vi "Master Setup Import.vi"(6 "Sorted Titles Indices":i32[](array[numeric]), 9 "Sorted Titles":string[](array[string]), 10 "Master Setup Path In":path, 11 "Master Setup In":path[](array[path])) -> (1 "Cancelled":bool, 2 "Master Setup Path Out":path, 3 "Master Setup Out":path[](array[path]))   [LabVIEW 2017]
uses:
  <vilib>/zip/NI_Unzip.lvlib
panel:
  out "Master Setup Assorted 2":path[](array[path])
  out "Tab Control":enum32{"Select Files", "Confirm Import"}(tab)
  in  "Files Available":i32[](listbox)
  in  "Files to Import":i32(listbox)
  in  "Remove":bool
  in  "Add":bool
  in  "Import":bool
  in  "Cancel":bool
  in  "Select File to Import From":path
  in  "Ok":bool
  in  "Cancel2":bool
  in  "Import All":bool
  in  "Auto Correct":bool
  out "Status":u16[](array[ring])
  out "Setup Files":string[](array[string])
  out "Target File Paths":path[](array[path])
  in  "Browse":bool[](array[boolean])
  # "REPS Import Setup Utility"
  # "File already Exists in the target path"
  # "File Path Ok"
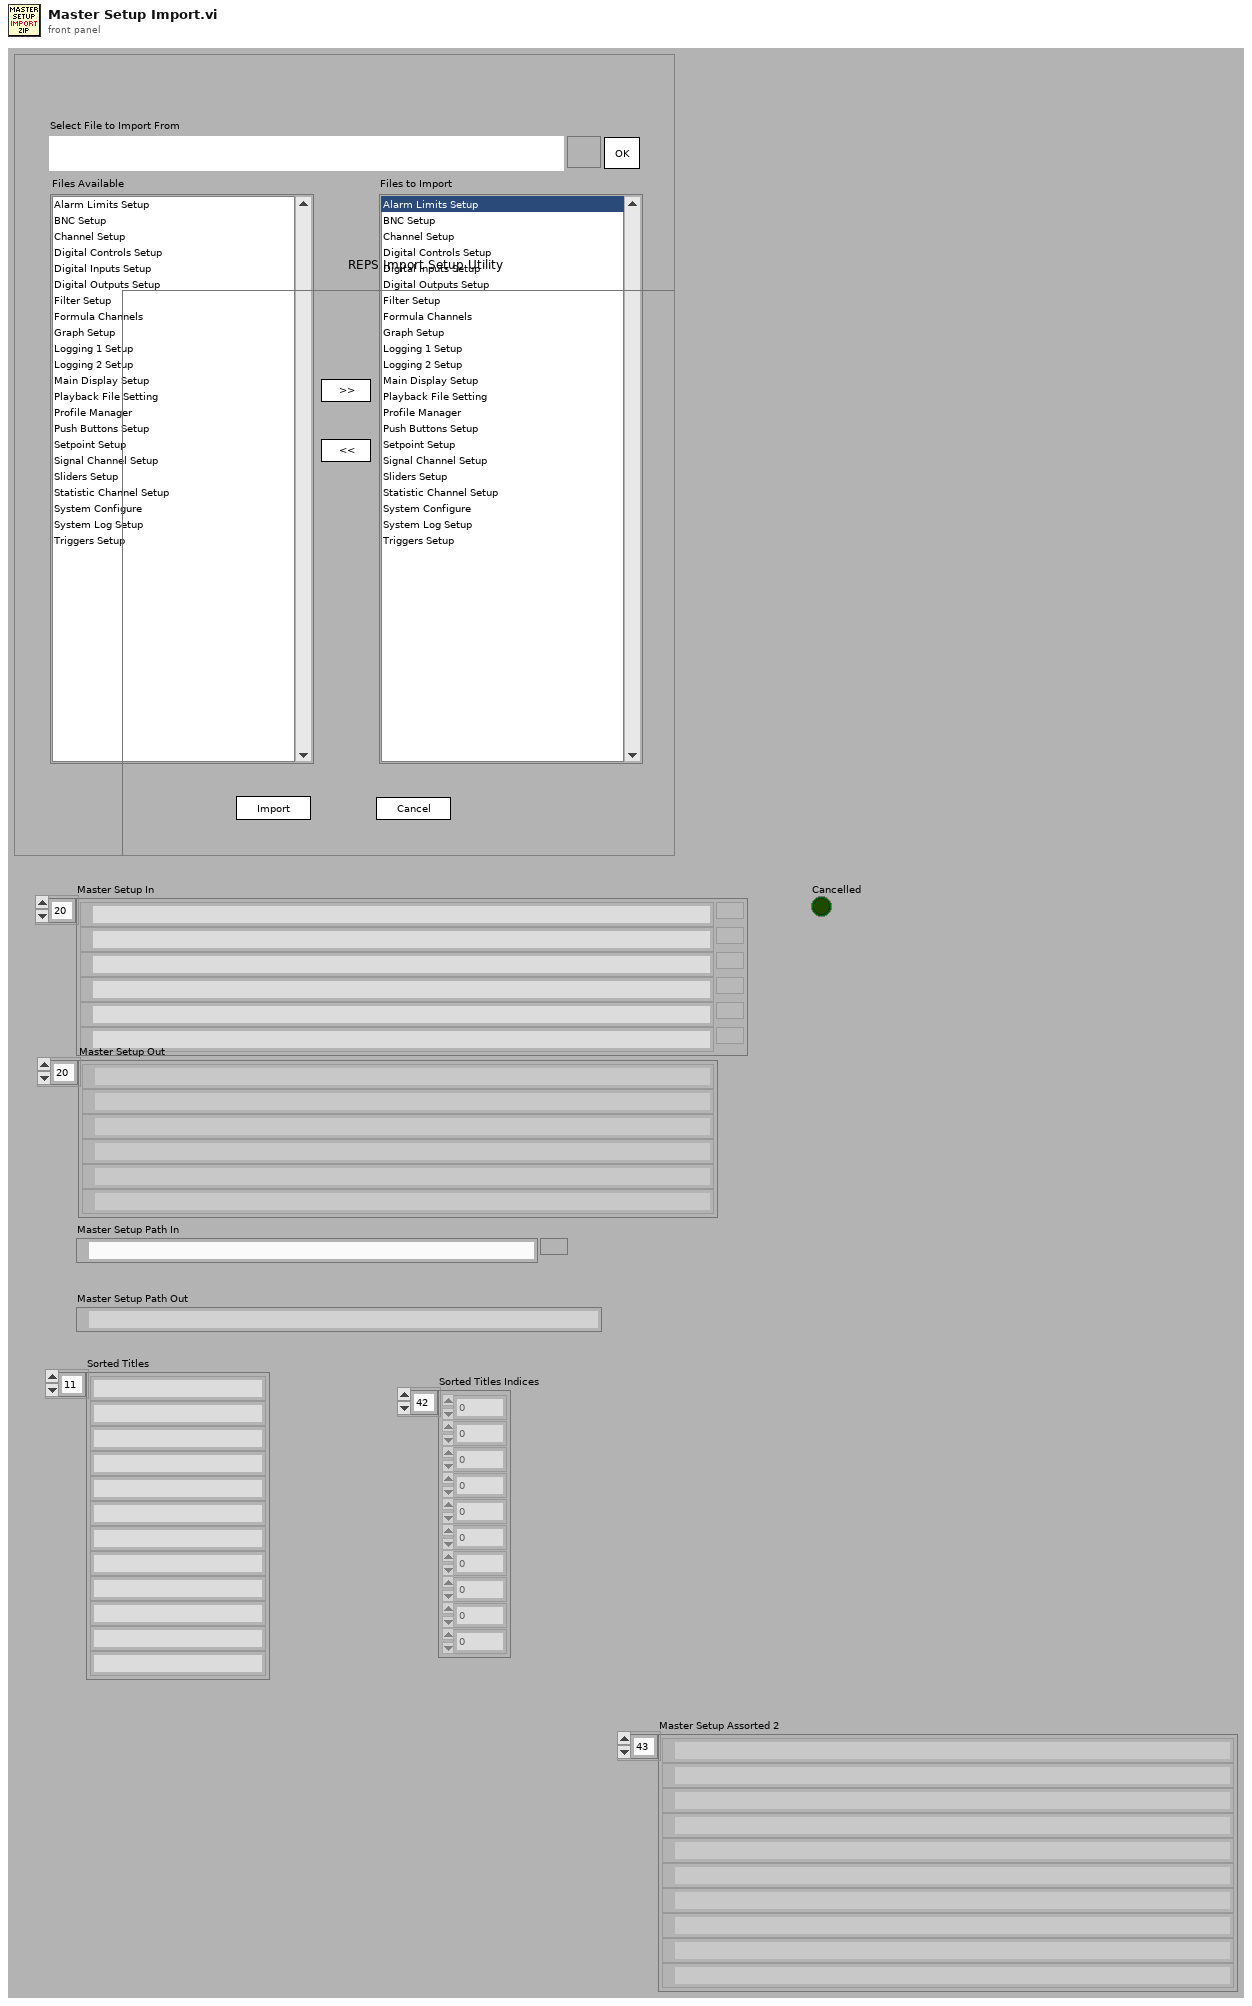
[diagram p1: front panel]
types:
  T1 = enum16{"<Init>", "<Poll>", "<Preview>", "<CheckFiles>", "<PopulateListBox>", "<ImportAddFile>", "<ImportRemoveFile>", "<Import>", "<CheckIfFileExists>", "<CopyFiles>", "<ConfirmOverwrite>", "<BrowseNewFile>", "<AutoCorrect>", "<Exit>"}
  T2 = enum32{"invalid app kind", "Development System", "Run Time System", "Student Edition", "Embedded LabVIEW", "Evaluation", "Custom"}
  T3 = enum8{"Enabled", "Disabled", "Disabled and Grayed Out"}
  T4 = cluster{"Preview files":path[], "Preview Folder":path, "File Types":string[], "Import files":path[], "Import File Types":string[], "Target files":path[], "Actual File Paths":path[], "vi reference":refnum<vi>, path[], "Sorted Titles":string[], i32[]}
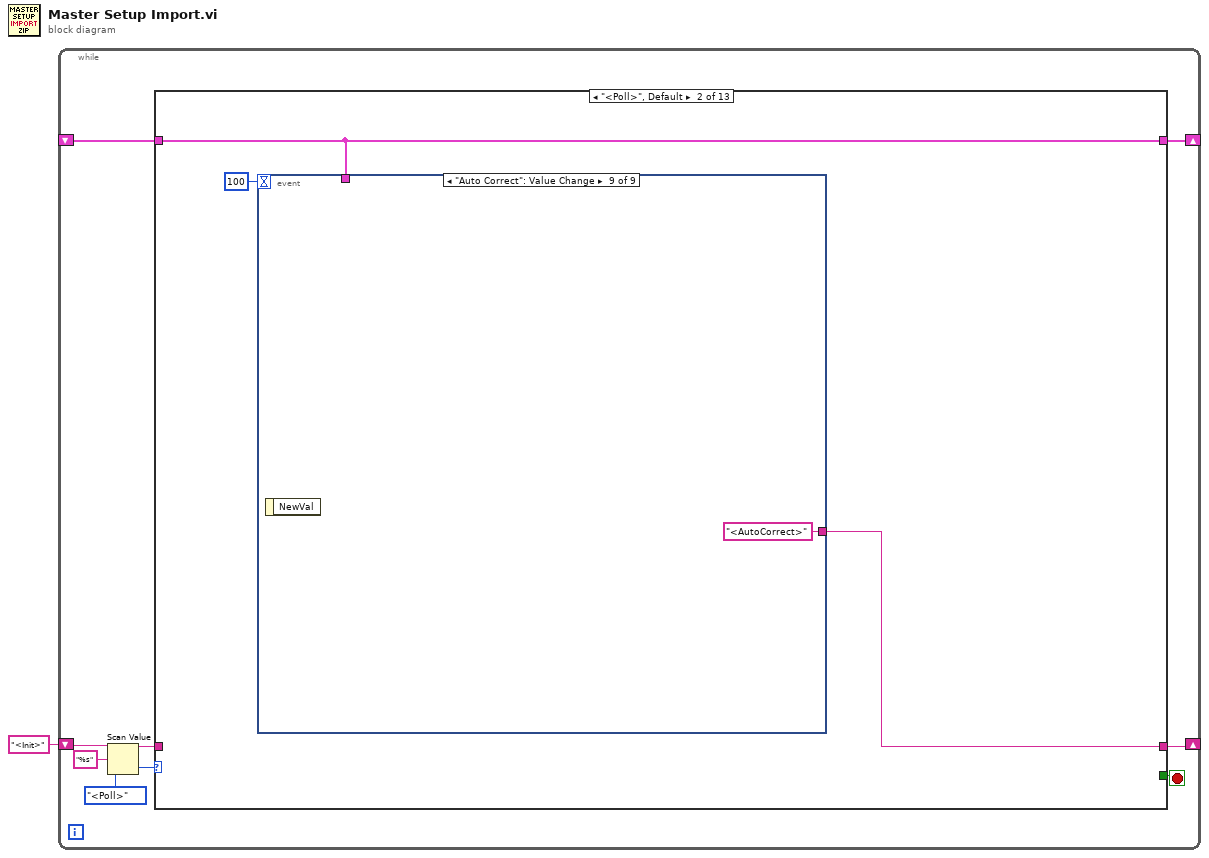
[diagram p0: block diagram]
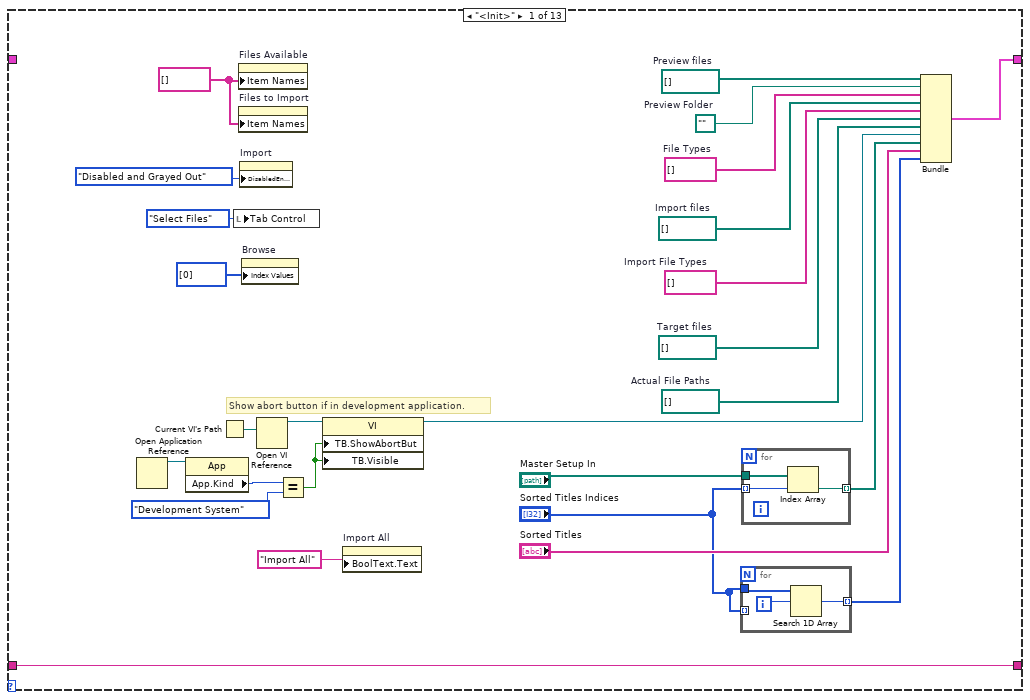
[diagram p2: hidden frame]
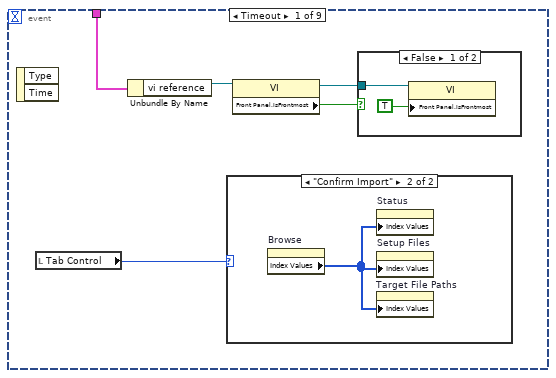
[diagram p3: hidden frame]
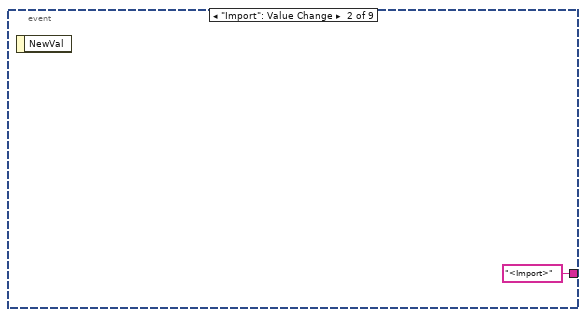
[diagram p6: hidden frame]
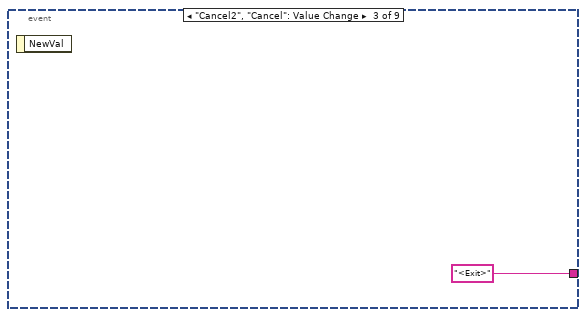
[diagram p7: hidden frame]
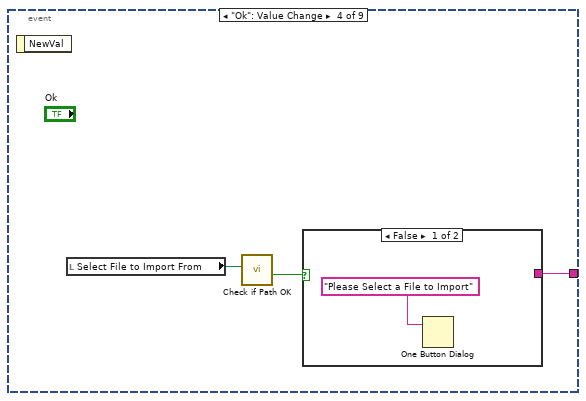
[diagram p8: hidden frame]
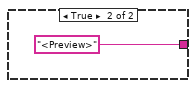
[diagram p9: hidden frame]
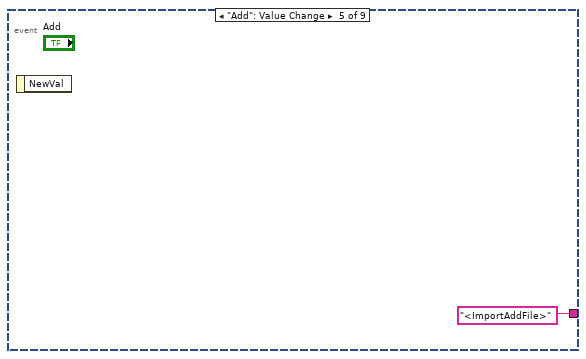
[diagram p10: hidden frame]
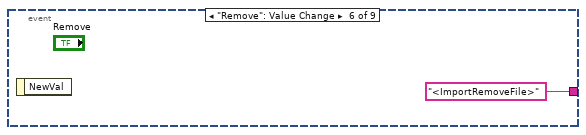
[diagram p11: hidden frame]
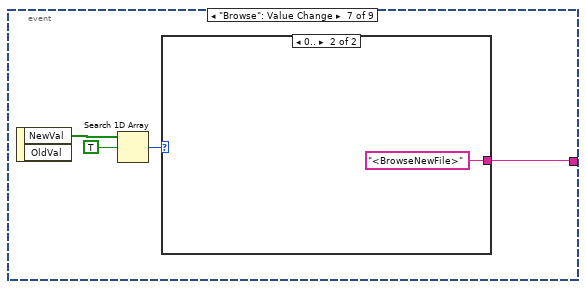
[diagram p12: hidden frame]
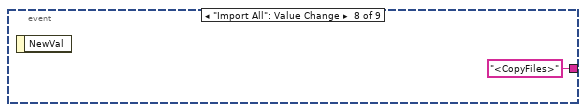
[diagram p14: hidden frame]
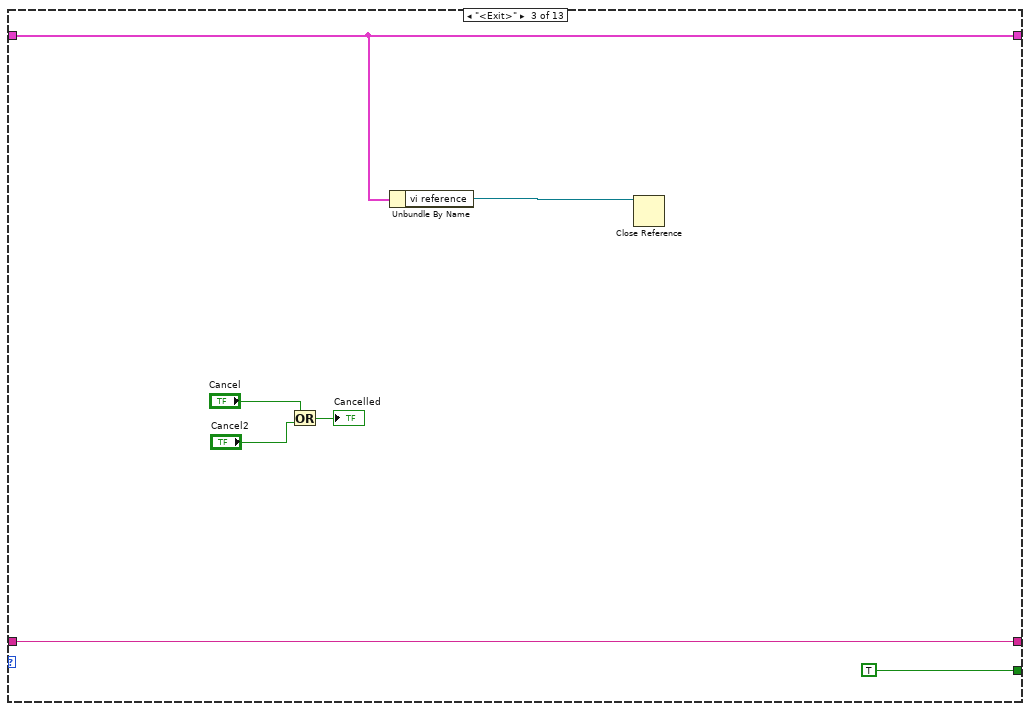
[diagram p15: hidden frame]
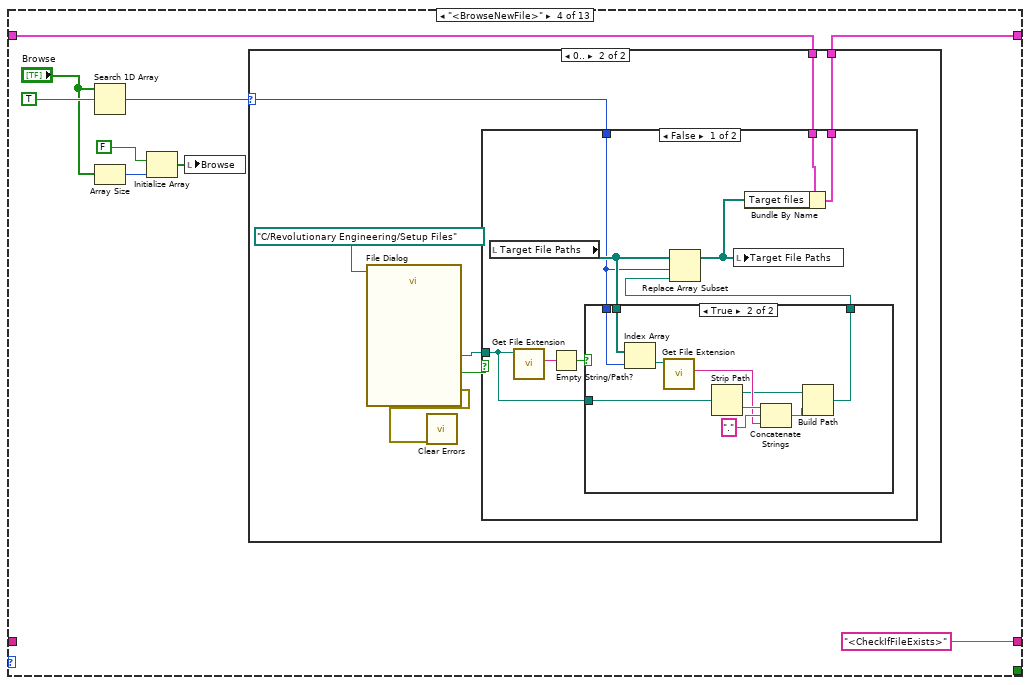
[diagram p16: hidden frame]
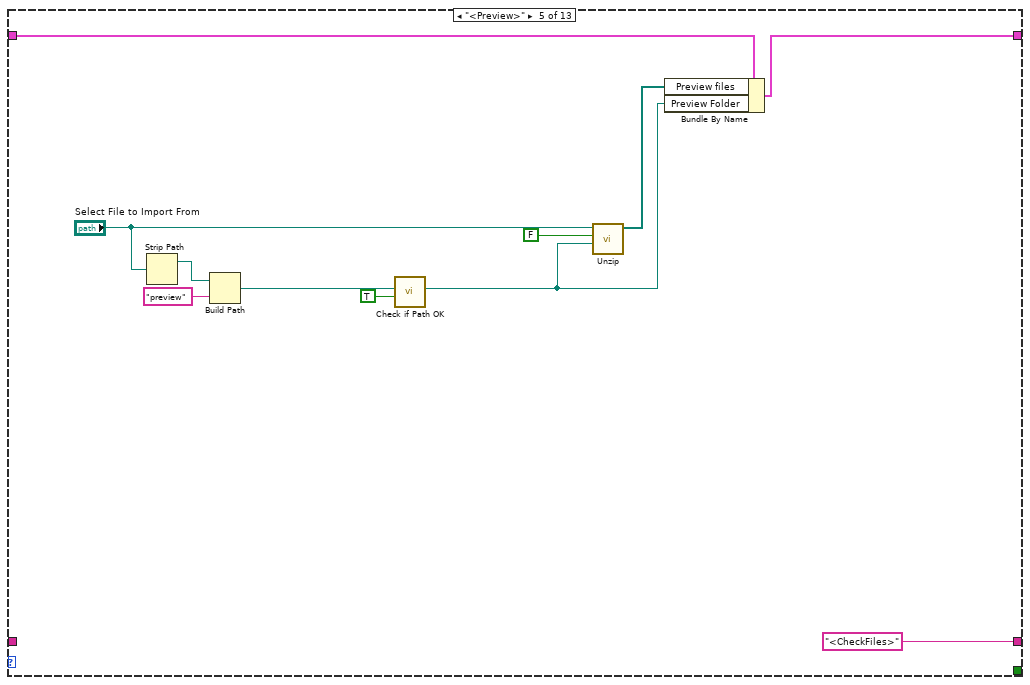
[diagram p20: hidden frame]
diagram:
  n1 = while {
    shift-right: [w8] -> _
    shift-left: "<Init>" -> [w10]
    shift-right: [w4] -> _
    shift-left: _ -> [w3]
    stop <- w5 stop-if-true
    n2 = Scan Value(string=w10, format string="%s", default (0 dbl)=T1."<Poll>") -> (output string=w9:string, value=w6:T1)
    n3 = case shown="\"<Poll>\", Default" w6 {
      tunnel: w9 -> [w34 _ w76 _ _ _ w157 w160 w180 _ _ _ _]
      tunnel: [w34 w44 w76 "<CheckIfFileExists>" "<CheckFiles>" w126 w157 w160 w180 "<CheckIfFileExists>" w220 "<Exit>" "<CheckIfFileExists>"] -> w8
      tunnel: [_ _ TRUE _ _ _ FALSE _ _ _ _ _ _] -> w5
      tunnel: [w33 w43 w74 w82 w122 w131 w147 w159 w181 w184 w224 w242 w278] -> w4
      tunnel: w3 -> [_ w43 w74 w83 w124 w131 w148 w159 w181 w185 w224 w242 w279]
      frame "<Init>" {
        w25 = path[] []  # Actual File Paths
        w26 = path[] []  # Target files
        w28 = string[] []  # Import File Types
        w29 = path[] []  # Import files
        w30 = string[] []  # File Types
        w31 = path ""  # Preview Folder
        w32 = path[] []  # Preview files
        w36 = string[] [] ("Item Names")
        # "Show abort button if in development application."
        n4 = Open Application Reference() -> (3:w24:refnum<vi>)  [unwired: 4 in, 1 out]
        n5 = property class="App"(reference=w24) -> ("App.Kind"=w23:T2)  [unwired: 1 in, 2 out]
        n6 = Current VI's Path() -> (path=w22:path)
        n7 = local write "Tab Control"(enum32{"Select Files", "Confirm Import"}."Select Files" ("Tab Control")) -> ()
        n8 = property on="Files Available" class="LstBox (strict)"("Item Names"=w36) -> ()  [unwired: 2 in, 2 out]
        n9 = property on="Files to Import" class="LstBox (strict)"("Item Names"=w36) -> ()  [unwired: 2 in, 2 out]
        n10 = property on="Import" class="Bool"("DisabledEnum"=T3."Disabled and Grayed Out" ("Disabled")) -> ()  [unwired: 2 in, 2 out]
        n11 = property on="Browse" class="Arr"("Index Values"=u32[] [0]) -> ()  [unwired: 2 in, 2 out]
        n12 = Open VI Reference(vi path=w22) -> (vi reference=w21:refnum<vi>)  [unwired: 5 in, 1 out]
        n13 = Equal?(x=w23, y=T2."Development System" ("Application:Kind")) -> (x = y?=w20:bool)
        n14 = property class="VI"(reference=w21, "TB.ShowAbortBut"=w20, "TB.Visible"=w20) -> (reference out=w18:refnum<vi>)  [unwired: 1 in, 1 out]
        n15 = property on="Import All" class="Bool"("BoolText.Text"="Import All" ("Label.Text")) -> ()  [unwired: 2 in, 2 out]
        n16 = for {
          tunnel: "Sorted Titles Indices" -> [w39]
          tunnel: "Sorted Titles Indices" -> [_] mode=indexing
          tunnel: [w37] -> w14 mode=indexing
          i -> [w38]
          n17 = Search 1D Array(1D array=w39, element=w38) -> (index of element=w37:i32)  [unwired: 1 in]
        }
        n18 = for {
          tunnel: "Master Setup In" -> [w42]
          tunnel: "Sorted Titles Indices" -> [w40] mode=indexing
          tunnel: [w41] -> w17 mode=indexing
          n19 = Index Array(array=w42, index=w40) -> (element=w41:path)
        }
        n20 = Bundle("Preview files"=w32, "Preview Folder"=w31, "File Types"=w30, "Import files"=w29, "Import File Types"=w28, "Target files"=w26, "Actual File Paths"=w25, "vi reference"=w18, w17, "Sorted Titles"="Sorted Titles", w14) -> (w33:T4)  [unwired: 1 in]
      }
      frame "<Poll>", Default {
        n21 = event shown="[8] \"Auto Correct\": Value Change" {
          selector: _ -> [_ _ _ _ _ _ _ _ _]
          dyn-events: _ -> [_ _ _ _ _ _ _ _ _]
          timeout: 100 -> [_ _ _ _ _ _ _ _ _]
          tunnel: [_ "<Import>" "<Exit>" w58 "<ImportAddFile>" "<ImportRemoveFile>" w63 "<CopyFiles>" "<AutoCorrect>"] -> w44
          tunnel: w43 -> [w49 _ _ _ _ _ _ _ _]
          event Timeout {
            n22 = event-data() -> ()  [unwired: 1 in, 2 out]
            n23 = local read "Tab Control"() -> (w50:enum32{"Select Files", "Confirm Import"})
            n24 = Unbundle By Name(w49) -> ("vi reference"=w48:refnum<vi>)
            n25 = case shown="\"Confirm Import\"" w50 {
              frame "Select Files", Default {
              }
              frame "Confirm Import" {
                n26 = property on="Browse" class="Arr"() -> ("Index Values"=w53:u32[])  [unwired: 2 in, 2 out]
                n27 = property on="Status" class="Arr (strict)"("Index Values"=w53) -> ()  [unwired: 2 in, 2 out]
                n28 = property on="Setup Files" class="Arr (strict)"("Index Values"=w53) -> ()  [unwired: 2 in, 2 out]
                n29 = property on="Target File Paths" class="Arr (strict)"("Index Values"=w53) -> ()  [unwired: 2 in, 2 out]
              }
            }
            n30 = property class="VI"(reference=w48) -> (reference out=w46:refnum<vi>, "Front Panel.IsFrontmost"=w47:bool)  [unwired: 1 in, 1 out]
            n31 = case shown="False" w47 {
              tunnel: w46 -> [w52 _]
              frame False {
                n32 = property class="VI"(reference=w52, "Front Panel.IsFrontmost"=TRUE ("Front Panel Window:Is Frontmost")) -> ()  [unwired: 1 in, 2 out]
              }
              frame True {
              }
            }
          }
          event "Import": Value Change {
            n33 = event-data() -> ()  [unwired: 1 in, 1 out]
          }
          event "Cancel2", "Cancel": Value Change {
            n34 = event-data() -> ()  [unwired: 1 in, 1 out]
          }
          event "Ok": Value Change {
            n35 = event-data() -> ()  [unwired: 1 in, 1 out]
            n36 = local read "Select File to Import From"() -> (w57:path)
            n37 = call "Check if Path OK.vi"("Path"=w57) -> ("Path OK"=w56:bool)  [unwired: 8 in, 2 out]
            n38 = case shown="False" w56 {
              tunnel: [_ "<Preview>"] -> w58
              frame False {
                n39 = One Button Dialog(message="Please Select a File to Import") -> ()  [unwired: 1 in, 1 out]
              }
              frame True {
              }
            }
          }
          event "Add": Value Change {
            n40 = event-data() -> ()  [unwired: 1 in, 1 out]
          }
          event "Remove": Value Change {
            n41 = event-data() -> ()  [unwired: 1 in, 1 out]
          }
          event "Browse": Value Change {
            n42 = event-data() -> ("NewVal"=w66:bool[])  [unwired: 1 in, 1 out]
            n43 = Search 1D Array(1D array=w66, element=TRUE) -> (index of element=w64:i32)  [unwired: 1 in]
            n44 = case shown="0.." w64 {
              tunnel: [_ "<BrowseNewFile>"] -> w63
              frame ..-1 {
              }
              frame 0.. {
              }
            }
          }
          event "Import All": Value Change {
            n45 = event-data() -> ()  [unwired: 1 in, 1 out]
          }
          event "Auto Correct": Value Change {
            n46 = event-data() -> ()  [unwired: 1 in, 1 out]
          }
        }
      }
      frame "<Exit>" {
        n47 = Or(x="Cancel", y="Cancel2") -> (x .or. y?=→"Cancelled":bool)
        n48 = Unbundle By Name(w74) -> ("vi reference"=w73:refnum<vi>)
        n49 = Close Reference(reference=w73) -> ()  [unwired: 1 in, 1 out]
      }
      frame "<BrowseNewFile>" {
        n50 = Search 1D Array(1D array="Browse", element=TRUE) -> (index of element=w84:i32)  [unwired: 1 in]
        n51 = Array Size(array="Browse") -> (size(s)=w80:i32)
        n52 = Initialize Array(FALSE ("element"), w80) -> (w78:bool[])
        n53 = local write "Browse"(w78) -> ()
        n54 = case shown="0.." w84 {
          selector: w84 -> [_ w90]
          tunnel: w83 -> [w86 w89]
          tunnel: [w86 w88] -> w82
          frame Default {
          }
          frame 0.. {
            n55 = call "File Dialog"("start path"=path "C:/Revolutionary Engineering/Setup Files") -> ("selected path"=w91:path, "cancelled"=w92:bool, "error out"=w87:errorcluster)  [unwired: 11 in, 1 out]
            n56 = call <vilib>:"Clear Errors.vi"("error in (no error)"=w87) -> ()  [unwired: 5 in, 2 out]
            n57 = case shown="False" w92 {
              tunnel: w91 -> [w95 _]
              tunnel: w90 -> [w96 _]
              tunnel: w89 -> [w102 w114]
              tunnel: [w101 w114] -> w88
              frame False {
                n58 = local read "Target File Paths"() -> (w97:path[])
                n59 = call <vilib>:"Get File Extension.vi"("file"=w95) -> ("lowercase file extension"=w99:string)  [unwired: 6 in, 4 out]
                n60 = Empty String/Path?(string/path=w99) -> (empty?=w98:bool)
                n61 = case shown="True" w98 {
                  tunnel: w97 -> [_ w113]
                  tunnel: w96 -> [_ w112]
                  tunnel: w95 -> [w103 w110]
                  tunnel: [w103 w104] -> w94
                  frame False {
                  }
                  frame True {
                    n62 = Index Array(array=w113, index=w112) -> (element=w111:path)
                    n63 = call <vilib>:"Get File Extension.vi"("file"=w111) -> ("lowercase file extension"=w107:string)  [unwired: 6 in, 4 out]
                    n64 = Strip Path(path=w110) -> (stripped path=w106:path, name=w109:string)
                    n65 = Concatenate Strings(w109, ".", w107) -> (w105:string)
                    n66 = Build Path(base path=w106, name or relative path=w105) -> (appended path=w104:path)
                  }
                }
                n67 = Replace Array Subset(array=w97, new element=w94, index=w96) -> (w100:path[])
                n68 = local write "Target File Paths"(w100) -> ()
                n69 = Bundle By Name(cluster=w102, "Target files"=w100) -> (w101:T4)
              }
              frame True {
              }
            }
          }
        }
      }
      frame "<Preview>" {
        n70 = Strip Path(path="Select File to Import From") -> (stripped path=w125:path)  [unwired: 1 out]
        n71 = Build Path(base path=w125, name or relative path="preview") -> (appended path=w116:path)
        n72 = call "Check if Path OK.vi"("Create if not found? (F)"=TRUE, "Path"=w116) -> ("Path"=w115:path)  [unwired: 7 in, 2 out]
        n73 = call <vilib>:"Unzip.vi"("Target directory (same as Zip file if empty)"=w115, "Preview only?"=FALSE, "Zip file"="Select File to Import From") -> ("Unzipped files"=w123:path[])  [unwired: 6 in, 2 out]
        n74 = Bundle By Name(cluster=w124, "Preview files"=w123, "Preview Folder"=w115) -> (w122:T4)
      }
      frame "<CheckFiles>" {
        n75 = Unbundle By Name(w131) -> ("Preview Folder"=w130:path)
        n76 = List Folder(path=w130) -> (filenames=w129:string[])  [unwired: 3 in, 3 out]
        n77 = Search 1D Array(1D array=w129, element="repsexport.txt") -> (index of element=w127:i32)  [unwired: 1 in]
        n78 = case shown="..-1" w127 {
          tunnel: ["<PopulateListBox>" "<Poll>"] -> w126
          frame 0.. {
            # "Valid REPS Export File"
            n79 = property on="Import" class="Bool"("DisabledEnum"=T3."Enabled" ("Disabled")) -> ()  [unwired: 2 in, 2 out]
          }
          frame ..-1 {
            # "Invalid REPS Export File"
            n80 = One Button Dialog(message="Invalid REPS Import File") -> ()  [unwired: 1 in, 1 out]
          }
        }
      }
      frame "<PopulateListBox>" {
        w140 = string[] []
        w138 = "," ("delimiter (Tab)")
        w139 = "%s" ("format string")
        n81 = Unbundle By Name(w148) -> ("Preview Folder"=w151:path)
        n82 = Build Path(base path=w151, name or relative path="repsexport.txt" ("element")) -> (appended path=w150:path)
        n83 = Open/Create/Replace File(file path (use dialog)=w150) -> (refnum out=w154:refnum<file>, error out=w155:errorcluster)  [unwired: 5 in, 1 out]
        n84 = Read from Text File(file (use dialog)=w154, error in=w155) -> (refnum out=w152:refnum<file>, text=w146:string, error out=w153:errorcluster)  [unwired: 2 in, 1 out]
        n85 = Close File(refnum=w152, error in=w153) -> ()  [unwired: 2 out]
        n86 = Match Pattern(string=w146, regular expression="REPS_File_Paths" ("string")) -> (before substring=w144:string, after substring=w143:string)  [unwired: 1 in, 2 out]
        n87 = Spreadsheet String To Array(delimiter (Tab)=w138, format string=w139, spreadsheet string=w144, array type (2D Dbl)=w140) -> (array=w137:string[])
        n88 = Spreadsheet String To Array(delimiter (Tab)=w138, format string=w139, spreadsheet string=w143, array type (2D Dbl)=w140) -> (array=w142:string[])
        n89 = for {
          tunnel: w137 -> [_] mode=indexing
          tunnel: [w158] -> w136 mode=indexing
          i -> [w158]
        }
        n90 = String To Path(string=w142) -> (path=w141:path[])
        n91 = property on="Files Available" class="LstBox (strict)"("Item Names"=w137, "Value"=w136) -> ()  [unwired: 2 in, 2 out]
        n92 = Bundle By Name(cluster=w148, "File Types"=w137, "Actual File Paths"=w141) -> (w147:T4)
      }
      frame "<ImportAddFile>" {
        n93 = property on="Files Available" class="LstBox (strict)"() -> ("Item Names"=w164:string[])  [unwired: 2 in, 2 out]
        n94 = property on="Files to Import" class="LstBox (strict)"() -> ("Item Names"=w162:string[])  [unwired: 2 in, 2 out]
        n95 = for {
          tunnel: "Files Available" -> [w169] mode=indexing
          tunnel: w164 -> [w170]
          shift-right: [w165] -> w161
          shift-left: w162 -> [w167]
          n96 = Index Array(array=w170, index=w169) -> (element=w166:string)
          n97 = Search 1D Array(1D array=w167, element=w166) -> (index of element=w168:i32)  [unwired: 1 in]
          n98 = case shown="..-1" w168 {
            tunnel: w167 -> [w171 w174]
            tunnel: w166 -> [_ w173]
            tunnel: [w171 w172] -> w165
            frame 0.. {
            }
            frame ..-1 {
              n99 = Build Array (concatenate)(w174, w173) -> (w172:string[])
            }
          }
        }
        n100 = property on="Files to Import" class="LstBox (strict)"("Item Names"=w161) -> ()  [unwired: 2 in, 2 out]
      }
      frame "<ImportRemoveFile>" {
        n101 = property on="Files to Import" class="LstBox (strict)"() -> ("Item Names"=w178:string[])  [unwired: 2 in, 2 out]
        n102 = Decrement(x="Files to Import") -> (x-1=w175:i32)
        n103 = Delete From Array(array=w178, length=1, index="Files to Import") -> (array with subset deleted=w177:string[])  [unwired: 1 out]
        n104 = local write "Files to Import"(w175) -> ()
        n105 = property on="Files to Import" class="LstBox (strict)"("Item Names"=w177) -> ()  [unwired: 2 in, 2 out]
      }
      frame "<Import>" {
        n106 = property on="Files to Import" class="LstBox (strict)"() -> ("Item Names"=w183:string[])  [unwired: 2 in, 2 out]
        n107 = Empty Array?(array=w183) -> (empty?=w182:bool)
        n108 = case shown="False" w182 {
          tunnel: w183 -> [w193 _]
          tunnel: w185 -> [w192 w205]
          tunnel: [w191 w205] -> w184
          frame False {
            n109 = Unbundle By Name(w192) -> ("Actual File Paths"=w189:path[], "Preview files"=w194:path[], "File Types"=w195:string[])
            n110 = for {
              tunnel: w193 -> [w203] mode=indexing
              tunnel: w195 -> [w200]
              tunnel: w194 -> [w202]
              tunnel: [w201] -> w190 mode=indexing
              tunnel: [w199] -> w187 mode=indexing
              tunnel: w189 -> [w198]
              tunnel: [w196] -> w188 mode=indexing
              n111 = Search 1D Array(1D array=w200, element=w203) -> (index of element=w197:i32)  [unwired: 1 in]
              n112 = Index Array(array=w198, index=w197) -> (element=w196:path)
              n113 = Index Array(array=w202, index=w197) -> (element=w201:path)
              n114 = Index Array(array=w200, index=w197) -> (element=w199:string)
            }
            n115 = Bundle By Name(cluster=w192, "Target files"=w188, "Import files"=w190, "Import File Types"=w187) -> (w191:T4)
          }
          frame True {
            n116 = One Button Dialog(message="No Files Selected for Import") -> ()  [unwired: 1 in, 1 out]
          }
        }
      }
      frame "<CheckIfFileExists>" {
        n117 = Unbundle By Name(w224) -> ("Target files"=w219:path[], "Import File Types"=w217:string[])
        "Target File Paths" <- w219
        "Setup Files" <- w217
        n118 = for {
          workers-P: _ -> [_]
          tunnel: w219 -> [w230] mode=indexing
          tunnel: [w228] -> w223 mode=indexing
          tunnel: [w225] -> w218 mode=indexing
          n119 = call "Check if Path OK.vi"("Create if not found? (F)"=FALSE, "Path"=w230) -> ("Path OK"=w228:bool)  [unwired: 7 in, 2 out]
          n120 = Select(t=u16 0 ("Ring"), s=w228, f=u16 2 ("Ring")) -> (s? t:f=w225:u16)
        }
        "Status" <- w218
        n121 = Array Size(array=w217) -> (size(s)=w210:i32)
        n122 = Initialize Array(FALSE, w210) -> (w212:bool[])
        n123 = Or Array Elements(Boolean array=w223) -> (logical OR=w208:bool)
        n124 = local write "Browse"(w212) -> ()
        n125 = Select(t="Replace All" ("Label.Text"), s=w208, f="Import All" ("Label.Text")) -> (s? t:f=w209:string)
        n126 = feedback #1(FALSE) -> (w216:bool)
        n127 = Or(x=w216, y=w208) -> (x .or. y?=w214:bool)
        n128 = feedback-in #1(w214) -> ()
        n129 = property on="Import All" class="Bool"("BoolText.Text"=w209) -> ()  [unwired: 2 in, 2 out]
        n130 = Select(t="<Poll>", s=w214, f="<CopyFiles>") -> (s? t:f=w220:string)
        "Tab Control" <- enum32{"Select Files", "Confirm Import"}."Confirm Import" ("Tab Control")
      }
      frame "<CopyFiles>" {
        n131 = Unbundle(w242) -> ("Import File Types"=w236:string[], w240:path[], "Sorted Titles"=w241:string[], w239:i32[])  [unwired: 7 out]
        n132 = Unbundle By Name(w242) -> ("Import files"=w247:path[], "Target files"=w246:path[])
        n133 = call <vilib>:"Clear Errors.vi"() -> ("error out"=w243:errorcluster)  [unwired: 6 in, 1 out]
        n134 = Search 1D Array(1D array=w236, element="Master Setup") -> (index of element=w234:i32)  [unwired: 1 in]
        n135 = for {
          tunnel: w247 -> [w275] mode=indexing
          tunnel: w246 -> [w268] mode=indexing
          shift-right: [w274] -> w244
          shift-left: w243 -> [w273]
          tunnel: [w272] -> w233 mode=indexing
          n136 = Strip Path(path=w268) -> (stripped path=w270:path)  [unwired: 1 out]
          n137 = call "Check if Path OK.vi"("Create if not found? (F)"=TRUE, "Path"=w270) -> ("error out"=w269:errorcluster)  [unwired: 7 in, 2 out]
          n138 = Copy(8:w269, 9:TRUE ("overwrite (F)"), 10:w268, 11:w275) -> (0:w266:errorcluster, 3:w272:path)  [unwired: 1 in, 1 out]
          n139 = Merge Errors(w266, w273) -> (w274:errorcluster)
        }
        n140 = for {
          tunnel: w236 -> [w259] mode=indexing
          tunnel: w241 -> [w260]
          shift-right: [w256] -> w237
          shift-left: w240 -> [w257]
          tunnel: w233 -> [w255] mode=indexing
          n141 = Search 1D Array(1D array=w260, element=w259) -> (index of element=w258:i32)  [unwired: 1 in]
          n142 = case shown="0.." w258 {
            selector: w258 -> [_ w263]
            tunnel: w257 -> [w261 w265]
            tunnel: [w261 w264] -> w256
            tunnel: w255 -> [_ w262]
            frame ..-1 {
            }
            frame 0.. {
              n143 = Replace Array Subset(array=w265, new element=w262, index=w263) -> (w264:path[])
            }
          }
        }
        "Master Setup Assorted 2" <- w237
        n144 = case shown="..-1" w234 {
          selector: w234 -> [_ w250]
          tunnel: w233 -> [_ w251]
          tunnel: [w248 w249] -> w232
          tunnel: "Master Setup Path In" -> [w248 _]
          frame ..-1 {
          }
          frame 0.. {
            n145 = Index Array(array=w251, index=w250) -> (element=w249:path)
          }
        }
        "Master Setup Path Out" <- w232
        n146 = for {
          tunnel: w237 -> [w254]
          tunnel: w239 -> [w252] mode=indexing
          tunnel: [w253] -> w238 mode=indexing
          n147 = Index Array(array=w254, index=w252) -> (element=w253:path)
        }
        "Master Setup Out" <- w238
        n148 = call <vilib>:"Simple Error Handler.vi"("error in (no error)"=w244) -> ()  [unwired: 4 in, 5 out]
      }
      frame "<AutoCorrect>" {
        n149 = Unbundle By Name(w279) -> ("Target files"=w280:path[])
        n150 = local read "Status"() -> (w281:u16[])
        n151 = for {
          tunnel: w281 -> [w284] mode=indexing
          tunnel: w280 -> [w283] mode=indexing
          tunnel: [w282] -> w277 mode=indexing
          n152 = case shown="0" w284 {
            tunnel: w283 -> [w285 w291]
            tunnel: [w285 w288] -> w282
            frame 2, Default {
              # "No Conflicts"
            }
            frame 0 {
              # "Conflicts"
              n153 = Format Date/Time String(time format string (%c)="%Y%m%d_%H%M%S") -> (date/time string=w294:string)  [unwired: 2 in]
              n154 = call <vilib>:"Get File Extension.vi"("file"=w291) -> ("filename without extension"=w287:string, "lowercase file extension"=w293:string)  [unwired: 6 in, 3 out]
              n155 = Strip Path(path=w291) -> (stripped path=w290:path)  [unwired: 1 out]
              n156 = Concatenate Strings(w287, " " ("string"), w294, "." ("time format string (%c)"), w293) -> (w289:string)
              n157 = Build Path(base path=w290, name or relative path=w289) -> (appended path=w288:path)
            }
          }
        }
        n158 = local write "Target File Paths"(w277) -> ()
        n159 = Bundle By Name(cluster=w279, "Target files"=w277) -> (w278:T4)
      }
    }
  }
